vi "Launch Host Reply Time Test Actor.vi"   [LabVIEW 2023]
uses:
  Host Reply Time Test Actor.lvclass
  C:/Program Files/National Instruments/LabVIEW 2023/vi.lib/ActorFramework/Actor/Actor.lvclass
  Host Reply Time Test Actor.lvclass/Host Reply Time Test Actor.ctl
  <vilib>/ni/Actors/Network Endpoint Actors/Protocols/Network Stream Strategy/Network Stream Initiator/Network Stream Initiator.lvclass
  C:/Program Files/National Instruments/LabVIEW 2023/vi.lib/ni/Actors/Network Endpoint Actors/Abstract Classes/Message Stream/Message Stream.lvclass
  <vilib>/ActorFramework/Actor/Actor.lvclass
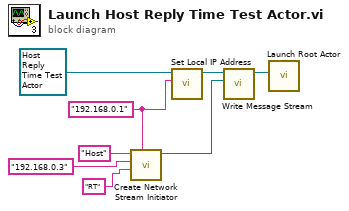
[diagram p0: block diagram]
diagram:
  w1 = "192.168.0.1" ("Local Address")
  n1 = call <vilib>:"Create Network Stream Initiator.vi"("Local Address"=w1, "Remote Name"="RT", "Remote Address"="192.168.0.3", "Name"="Host") -> ("Network Stream Initiator out"=w3:refnum<class "Network Stream Initiator.lvclass">)  [unwired: 7 in]
  n2 = call "Set Local IP Address.vi"("Local IP Address"=w1, "Host Reply Time Test Actor in"=refnum<class "Host Reply Time Test Actor.lvclass"> refnum ("Host Reply Time Test Actor.lvlib:Host Reply Time Test Actor.lvclass")) -> ("Host Reply Time Test Actor out"=w2:refnum<class "Host Reply Time Test Actor.lvclass">)  [unwired: 9 in]
  n3 = call "Write Message Stream.vi"("Message Stream.lvclass"=w3, "Host Reply Time Test Actor in"=w2) -> ("Host Reply Time Test Actor out"=w4:refnum<class "Host Reply Time Test Actor.lvclass">)  [unwired: 8 in, 1 out]
  n4 = call <vilib>:"Launch Root Actor.vi"("Actor"=w4) -> ()  [unwired: 9 in, 2 out]
